vi "Copy Image for buffer.vi"(11 "Refnum in":T1) -> (0 "error out":errorcluster, 2 "Image Name":string, 3 "Refnum out":T1)   [LabVIEW 2020]
uses:
  <vilib>/vision/Image Controls.llb/IMAQ Image.ctl
panel:
  out "error out 8":errorcluster
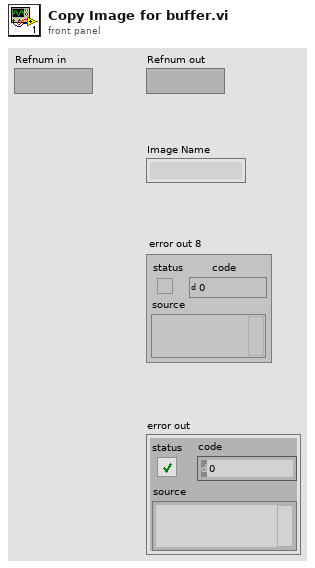
[diagram p1: front panel]
types:
  T1 = typedef "IMAQ Image.ctl" = refnum<image>
  T2 = typedef "Image Type" = u32
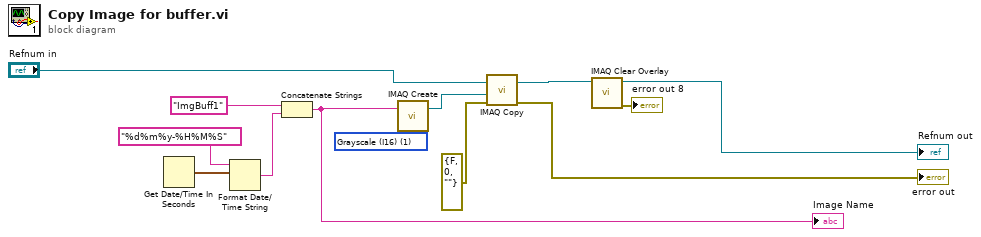
[diagram p0: block diagram]
diagram:
  w1 = T2 1 items=["Grayscale (U8)", "Grayscale (I16)", "Grayscale (SGL)", "Complex (CSG)", "RGB (U32)", "HSL (U32)", "RGB (U64)", "Grayscale (U16)"] ("Image Type")
  n1 = Get Date/Time In Seconds() -> (seconds since 1Jan1904=w6:timestamp)
  n2 = Format Date/Time String(time format string (%c)="%d%m%y-%H%M%S", seconds (now)=w6) -> (date/time string=w8:string)  [unwired: 1 in]
  n3 = Concatenate Strings("ImgBuff1" ("Image Name"), w8) -> (w13:string)
  "Image Name" <- w13
  n4 = call "IMAQ Create"("Image Name"=w13, "Image Type"=w1) -> ("New Image"=w2:T1)  [unwired: 3 in, 1 out]
  n5 = call "IMAQ Copy"("error in (no error)"=errorcluster {"status"=FALSE, "code"=0, "source"=""}, "Image Dst"=w2, "Image Src"="Refnum in") -> ("error out"=→"error out":errorcluster, "Image Dst Out"=w9:T1)  [unwired: 3 in]
  n6 = call "IMAQ Clear Overlay"("Image"=w9) -> ("error out"=→"error out 8":errorcluster, "Image Out"=→"Refnum out":T1)  [unwired: 9 in]
